vi "Question Prompt Display.vi"(8 "error in (no error)":errorcluster, 9 "Image Path":path, 10 "Prompt":string="A boolean text will center vertically and horizontally but won't word wrap", 11 "Controller in":refnum<class "Controller.lvclass">) -> (0 "error out":errorcluster, 3 "Controller out":refnum<class "Controller.lvclass">)   [LabVIEW 2024, in "Controller.lvlib" / "Controller.lvclass"]
uses:
  Controller.lvclass
  Controller.lvclass/Controller.ctl
  <vilib>/Dataflow_G/G-Image/Image IO/Polymorphic VIs/Load Image (Path).vi
  <vilib>/Dataflow_G/G-Image/G-Image.lvlib
panel:
  out "2D Picture":picture
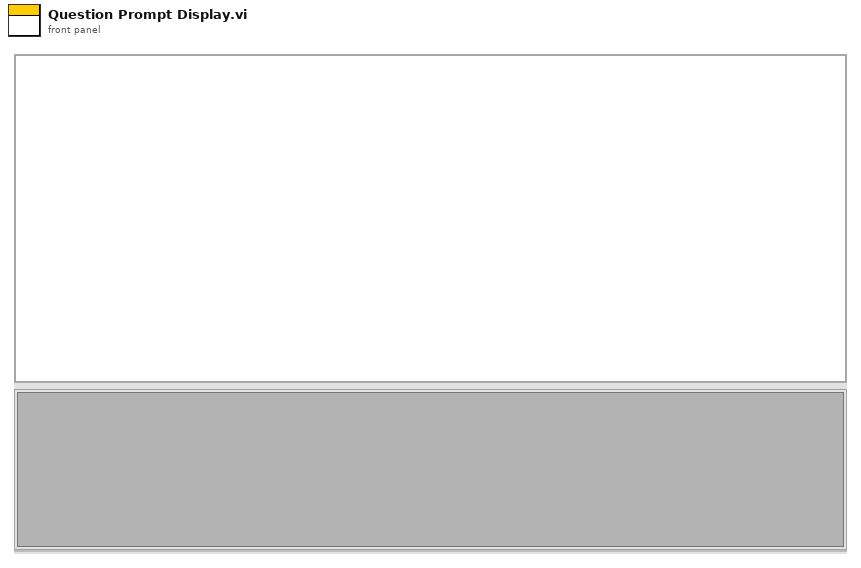
[diagram p1: front panel]
types:
  T1 = typedef "imagedata.ctl" = cluster{"image type":i32, "image depth":i32, "image":u8[], "mask":u8[], "colors":u32[], "Rectangle":cluster{"left":i16, "top":i16, "right":i16, "bottom":i16}}
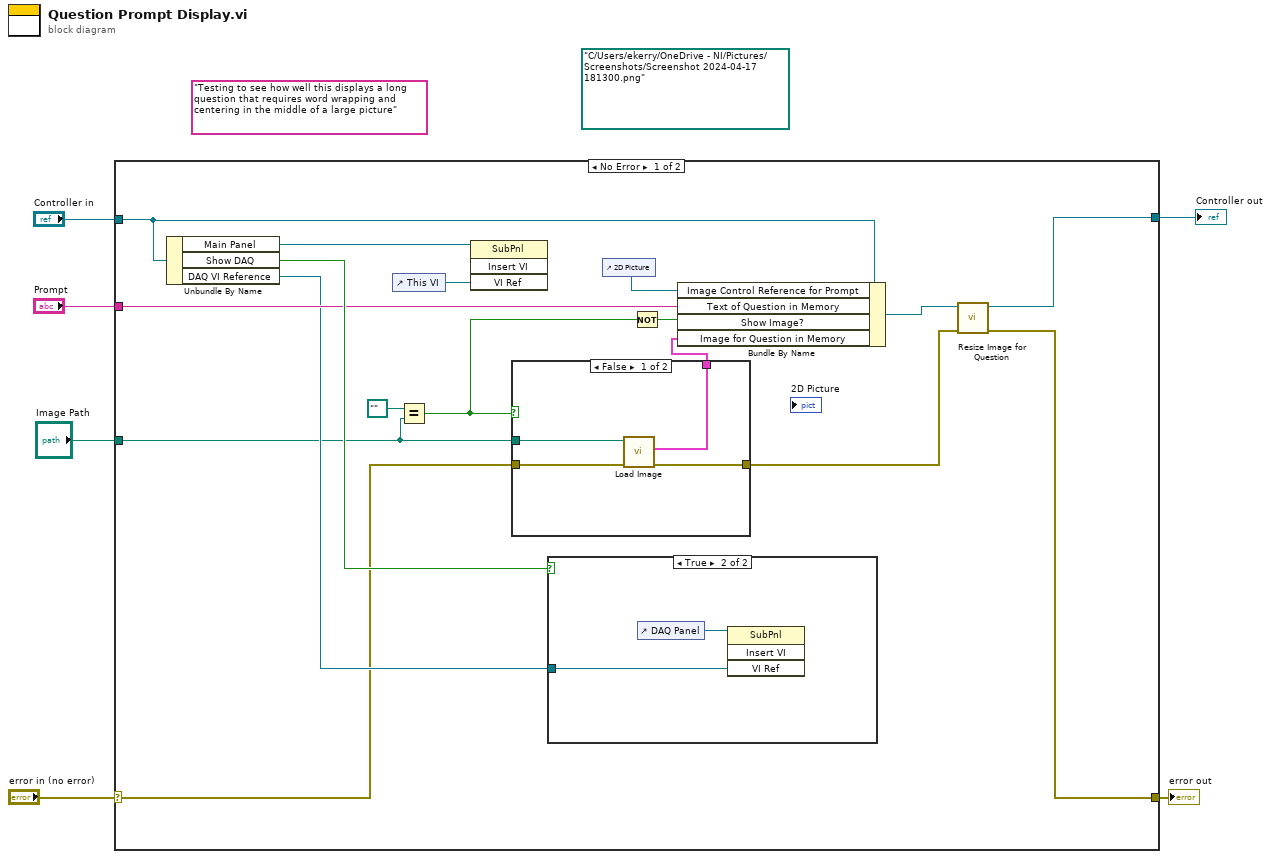
[diagram p0: block diagram]
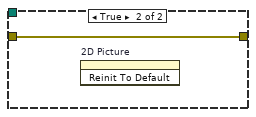
[diagram p2: hidden frame]
diagram:
  (unwired) path "C:/Users/ekerry/OneDrive - NI/Pictures/Screenshots/Screenshot 2024-04-17 181300.png" ("Path")
  (unwired) "Testing to see how well this displays a long question that requires word wrapping and centering in the middle of a large picture" ("text")
  n1 = case shown="No Error" "error in (no error)" {
    selector: "error in (no error)" -> [w13 w32]
    tunnel: [w20 w32] -> w5
    tunnel: [w18 w31] -> w3
    tunnel: "Controller in" -> [w21 w31]
    tunnel: "Prompt" -> [w15 _]
    tunnel: "Image Path" -> [w11 _]
    frame No Error {
      n2 = Unbundle By Name(w21) -> ("Main Panel"=w23:refnum<vi>, "Show DAQ"=w16:bool, "DAQ VI Reference"=w14:refnum<vi>)
      n3 = control-ref of="This VI"() -> (w22:refnum<vi>)
      n4 = Equal?(x=path "", y=w11) -> (x = y?=w8:bool)
      n5 = invoke on="Invoke Node" class="SubPnl" method="Insert VI"(reference=w23, "VI Ref"=w22) -> ()  [unwired: 2 in, 4 out]
      n6 = case shown="False" w8 {
        tunnel: [w27 _] -> w7
        tunnel: w13 -> [w26 w28]
        tunnel: [w25 w28] -> w12
        tunnel: w11 -> [w24 _]
        frame False {
          n7 = call-poly <vilib>:"Load Image.vi"("error in (no error)"=w26, "Path In"=w24) -> ("error out"=w25:errorcluster, "Image"=w27:T1)  [unwired: 7 in, 1 out]
        }
        frame True {
          n8 = invoke on="2D Picture" class="Pict" method="Reinit To Default"() -> ()  [unwired: 3 in, 3 out]
        }
      }
      n9 = case shown="True" w16 {
        tunnel: w14 -> [_ w29]
        frame False {
        }
        frame True {
          n10 = control-ref of="DAQ Panel"() -> (w30:refnum<vi>)
          n11 = invoke on="Invoke Node" class="SubPnl" method="Insert VI"(reference=w30, "VI Ref"=w29) -> ()  [unwired: 2 in, 4 out]
        }
      }
      n12 = control-ref of="2D Picture"() -> (w17:refnum<vi>)
      n13 = Not(x=w8) -> (.not. x?=w9:bool)
      n14 = Bundle By Name(cluster=w21, "Image Control Reference for Prompt"=w17, "Text of Question in Memory"=w15, "Show Image?"=w9, "Image for Question in Memory"=w7) -> (w19:refnum<class "Controller.lvclass">)
      n15 = call-dynamic "Resize Image for Question.vi"("error in (no error)"=w12, "Controller in"=w19) -> ("error out"=w20:errorcluster, "Controller Out"=w18:refnum<class "Controller.lvclass">)  [unwired: 8 in]
    }
    frame Error {
    }
  }
  "error out" <- w5
  "Controller out" <- w3
